vi "SMTPSimple.vi"(8 "错误输入（无错误）":errorcluster, 9 "body":string, 11 "mail info":T1={"host"="smtp-mail.outlook.com", "port"=587, "username"="", "password"="", "From"="", "to"="", "subject"=""}) -> (0 "error out":errorcluster)   [LabVIEW 2017]
panel:
  in  "IsBodyHtml":bool=TRUE
  in  "EnableSSl":bool=TRUE
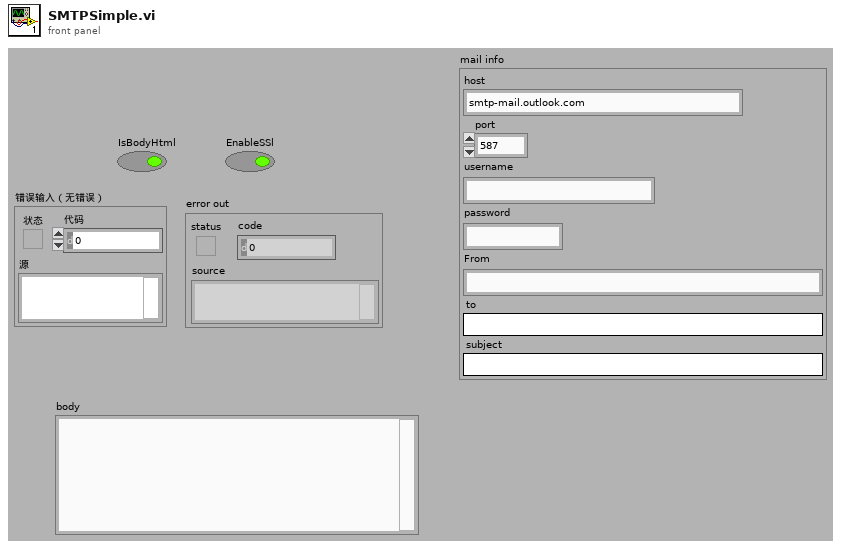
[diagram p1: front panel]
types:
  T1 = cluster{"host":string, "port":i32, "username":string, "password":string, "From":string, "to":string, "subject":string}
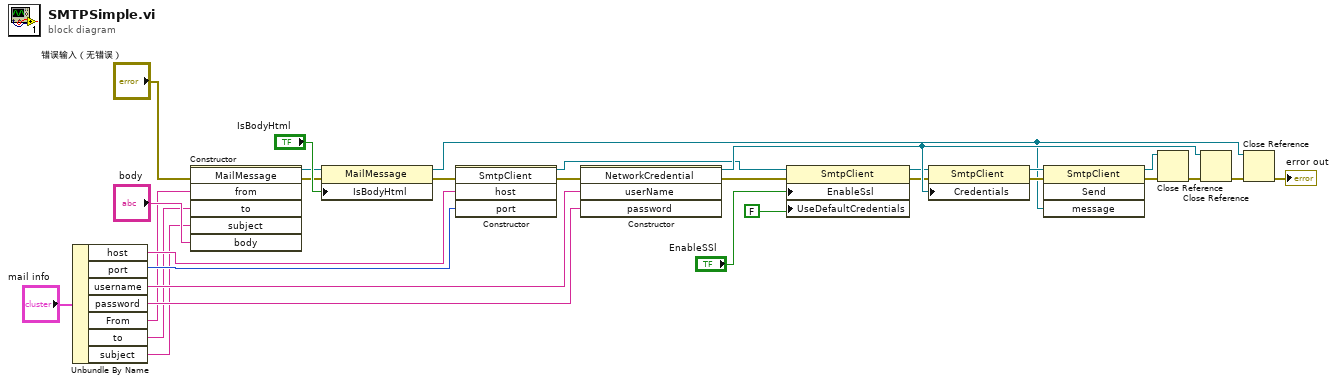
[diagram p0: block diagram]
diagram:
  n1 = Unbundle By Name("mail info") -> ("host"=w7:string, "port"=w6:i32, "username"=w5:string, "password"=w4:string, "From"=w3:string, "to"=w2:string, "subject"=w1:string)
  n2 = constructor class="MailMessage"(error in="错误输入（无错误）", "from"=w3, "to"=w2, "subject"=w1, "body"="body") -> (reference out=w14:refnum<k24>, error out=w12:errorcluster)  [unwired: 2 in, 5 out]
  n3 = property class="MailMessage"(reference=w14, error in=w12, "IsBodyHtml"="IsBodyHtml") -> (reference out=w13:refnum<k24>, error out=w10:errorcluster)
  n4 = constructor class="SmtpClient"(error in=w10, "host"=w7, "port"=w6) -> (reference out=w23:refnum<k24>, error out=w25:errorcluster)  [unwired: 2 in, 3 out]
  n5 = constructor class="NetworkCredential"(error in=w25, "userName"=w5, "password"=w4) -> (reference out=w28:refnum<k24>, error out=w24:errorcluster)  [unwired: 2 in, 3 out]
  n6 = property class="SmtpClient"(reference=w23, error in=w24, "EnableSsl"="EnableSSl", "UseDefaultCredentials"=FALSE) -> (reference out=w22:refnum<k24>, error out=w21:errorcluster)
  n7 = property class="SmtpClient"(reference=w22, error in=w21, "Credentials"=w28) -> (reference out=w17:refnum<k24>, error out=w16:errorcluster)
  n8 = invoke class="SmtpClient" method="Send"(reference=w17, error in=w16, "message"=w13) -> (reference out=w20:refnum<k24>, error out=w19:errorcluster)  [unwired: 1 in, 2 out]
  n9 = Close Reference(reference=w20, error in (no error)=w19) -> (error out=w27:errorcluster)
  n10 = Close Reference(reference=w28, error in (no error)=w27) -> (error out=w26:errorcluster)
  n11 = Close Reference(reference=w13, error in (no error)=w26) -> (error out=→"error out":errorcluster)
